vi "TCS_CFN_VS50BR_v1.vi"() -> ()   [LabVIEW 2017]
uses:
  <vilib>/Instr/_visa.llb/VISA Configure Serial Port (Instr).vi
panel:
  in  "Tab Control 4":enum32{"TCS_Utility", "TCS_Utility 2"}(tab)
  in  "Fact Reserved":bool
  in  "Download":bool
  in  "Fact Config":bool
  in  "NavOn":bool
  in  "Init":bool
  out "Half Second":bool[][](array[boolean])=[[FALSE, FALSE, FALSE, FALSE, FALSE, FALSE, FALSE, FALSE, FALSE, FALSE], [FALSE, FALSE, TRUE, TRUE, TRUE, TRUE, TRUE, FALSE, FALSE, FALSE], [FALSE, TRUE, FALSE, FALSE, FALSE, FALSE, FALSE, TRUE, FALSE, FALSE], [FALSE, TRUE, FALSE, FALSE, FALSE, FALSE, FALSE, TRUE, FALSE, FALSE], [FALSE, TRUE, FALSE, FALSE, FALSE, FALSE, FALSE, TRUE, FALSE, FALSE], [FALSE, TRUE, FALSE, FALSE, FALSE, FALSE, FALSE, TRUE, FALSE, FALSE], [FALSE, TRUE, FALSE, FALSE, FALSE, FALSE, FALSE, TRUE, FALSE, FALSE], [FALSE, TRUE, FALSE, FALSE, FALSE, FALSE, FALSE, TRUE, FALSE, FALSE], [FALSE, FALSE, TRUE, TRUE, TRUE, TRUE, TRUE, FALSE, FALSE, FALSE], [FALSE, FALSE, FALSE, FALSE, FALSE, FALSE, FALSE, FALSE, FALSE, FALSE]]
  out "Min 1":bool[][](array[boolean])=[[FALSE, FALSE, FALSE, FALSE, FALSE, FALSE, FALSE, FALSE, FALSE, FALSE], [FALSE, FALSE, TRUE, TRUE, TRUE, TRUE, TRUE, FALSE, FALSE, FALSE], [FALSE, TRUE, FALSE, FALSE, FALSE, FALSE, FALSE, TRUE, FALSE, FALSE], [FALSE, TRUE, FALSE, FALSE, FALSE, FALSE, FALSE, TRUE, FALSE, FALSE], [FALSE, TRUE, FALSE, FALSE, FALSE, FALSE, FALSE, TRUE, FALSE, FALSE], [FALSE, TRUE, FALSE, FALSE, FALSE, FALSE, FALSE, TRUE, FALSE, FALSE], [FALSE, TRUE, FALSE, FALSE, FALSE, FALSE, FALSE, TRUE, FALSE, FALSE], [FALSE, TRUE, FALSE, FALSE, FALSE, FALSE, FALSE, TRUE, FALSE, FALSE], [FALSE, FALSE, TRUE, TRUE, TRUE, TRUE, TRUE, FALSE, FALSE, FALSE], [FALSE, FALSE, FALSE, FALSE, FALSE, FALSE, FALSE, FALSE, FALSE, FALSE]]
  out "Min 0":bool[][](array[boolean])=[[FALSE, FALSE, FALSE, FALSE, FALSE, FALSE, FALSE, FALSE, FALSE, FALSE], [FALSE, FALSE, TRUE, TRUE, TRUE, TRUE, TRUE, FALSE, FALSE, FALSE], [FALSE, TRUE, FALSE, FALSE, FALSE, FALSE, FALSE, TRUE, FALSE, FALSE], [FALSE, TRUE, FALSE, FALSE, FALSE, FALSE, FALSE, TRUE, FALSE, FALSE], [FALSE, TRUE, FALSE, FALSE, FALSE, FALSE, FALSE, TRUE, FALSE, FALSE], [FALSE, TRUE, FALSE, FALSE, FALSE, FALSE, FALSE, TRUE, FALSE, FALSE], [FALSE, TRUE, FALSE, FALSE, FALSE, FALSE, FALSE, TRUE, FALSE, FALSE], [FALSE, TRUE, FALSE, FALSE, FALSE, FALSE, FALSE, TRUE, FALSE, FALSE], [FALSE, FALSE, TRUE, TRUE, TRUE, TRUE, TRUE, FALSE, FALSE, FALSE], [FALSE, FALSE, FALSE, FALSE, FALSE, FALSE, FALSE, FALSE, FALSE, FALSE]]
  out "Hour 1":bool[][](array[boolean])=[[FALSE, FALSE, FALSE, FALSE, FALSE, FALSE, FALSE, FALSE, FALSE, FALSE], [FALSE, FALSE, TRUE, TRUE, TRUE, TRUE, TRUE, FALSE, FALSE, FALSE], [FALSE, TRUE, FALSE, FALSE, FALSE, FALSE, FALSE, TRUE, FALSE, FALSE], [FALSE, TRUE, FALSE, FALSE, FALSE, FALSE, FALSE, TRUE, FALSE, FALSE], [FALSE, TRUE, FALSE, FALSE, FALSE, FALSE, FALSE, TRUE, FALSE, FALSE], [FALSE, TRUE, FALSE, FALSE, FALSE, FALSE, FALSE, TRUE, FALSE, FALSE], [FALSE, TRUE, FALSE, FALSE, FALSE, FALSE, FALSE, TRUE, FALSE, FALSE], [FALSE, TRUE, FALSE, FALSE, FALSE, FALSE, FALSE, TRUE, FALSE, FALSE], [FALSE, FALSE, TRUE, TRUE, TRUE, TRUE, TRUE, FALSE, FALSE, FALSE], [FALSE, FALSE, FALSE, FALSE, FALSE, FALSE, FALSE, FALSE, FALSE, FALSE]]
  out "Hour 0":bool[][](array[boolean])=[[FALSE, FALSE, FALSE, FALSE, FALSE, FALSE, FALSE, FALSE, FALSE, FALSE], [FALSE, FALSE, TRUE, TRUE, TRUE, TRUE, TRUE, FALSE, FALSE, FALSE], [FALSE, TRUE, FALSE, FALSE, FALSE, FALSE, FALSE, TRUE, FALSE, FALSE], [FALSE, TRUE, FALSE, FALSE, FALSE, FALSE, FALSE, TRUE, FALSE, FALSE], [FALSE, TRUE, FALSE, FALSE, FALSE, FALSE, FALSE, TRUE, FALSE, FALSE], [FALSE, TRUE, FALSE, FALSE, FALSE, FALSE, FALSE, TRUE, FALSE, FALSE], [FALSE, TRUE, FALSE, FALSE, FALSE, FALSE, FALSE, TRUE, FALSE, FALSE], [FALSE, TRUE, FALSE, FALSE, FALSE, FALSE, FALSE, TRUE, FALSE, FALSE], [FALSE, FALSE, TRUE, TRUE, TRUE, TRUE, TRUE, FALSE, FALSE, FALSE], [FALSE, FALSE, FALSE, FALSE, FALSE, FALSE, FALSE, FALSE, FALSE, FALSE]]
  in  "Stop":bool
  out "string in":string
  out "string out":string
  out "DV_Word":bool[](array[boolean])
  out "B_55":u8 format="%x"
  out "B_54":u8 format="%x"
  out "String":string
  in  "Send":bool
  in  "Tab Control":enum32{"Page 1", "Page 2", "Page 3"}(tab)
  in  "Offset Yaw":sgl(slide) scale=-180.0..180.0
  in  "Offset Roll":sgl(slide) scale=-180.0..180.0
  in  "Offset Pitch":sgl(slide) scale=-180.0..180.0
  in  "Longitude":sgl(slide)=-45.860622 scale=-180.0..180.0
  in  "Latitude":sgl(slide)=-23.213156 scale=-90.0..90.0
  in  "Azimuth":sgl(slide) scale=0.0..360.0
  in  "Height":sgl(slide)=622.367 scale=-2000.0..10000.0
  in  "LP_X-Up":sgl(slide) scale=-180.0..180.0
  in  "LP_Y-Easth":sgl(slide)=0.128098 scale=-180.0..180.0
  in  "LP_Z-North":sgl(slide)=0.467339 scale=-180.0..180.0
  # "B#55 (Configuration and Command Mode)"
  # "0x35"
  # "0xBD"
  # "0XFA"
  # "0XEE"
  # "0XAB"
  # "B#54 (Data Validity Word)"
  # "1= Installation Offset input valid data\n1= Launch Azimuth geodetic orientation, position, (lat, long, height) valid \n1= Velocity input valid data \nRFU\nRFU\nRFU\n 7,6     00= \"Init Cmd\" (Configuration parameters setting)\n           10= \"NAV_On\"\n           01= Reserved\n           11= Enter Configuration Mode"
  # "0\n1\n2\n3\n4\n5\n6\n7"
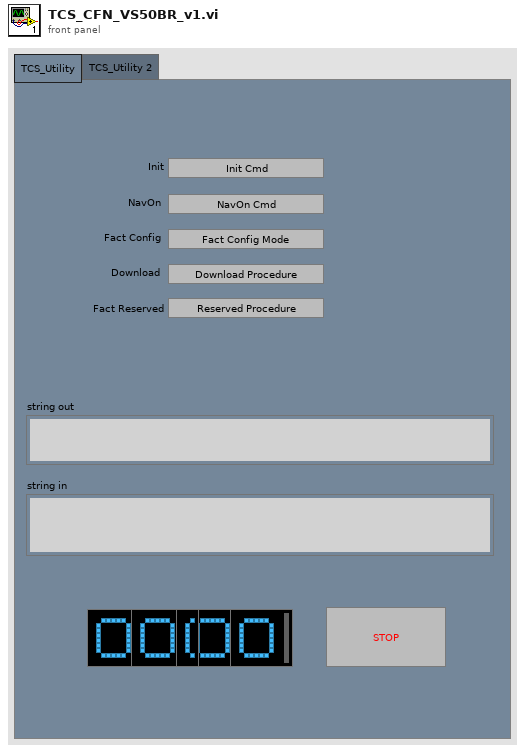
[diagram p1: front panel]
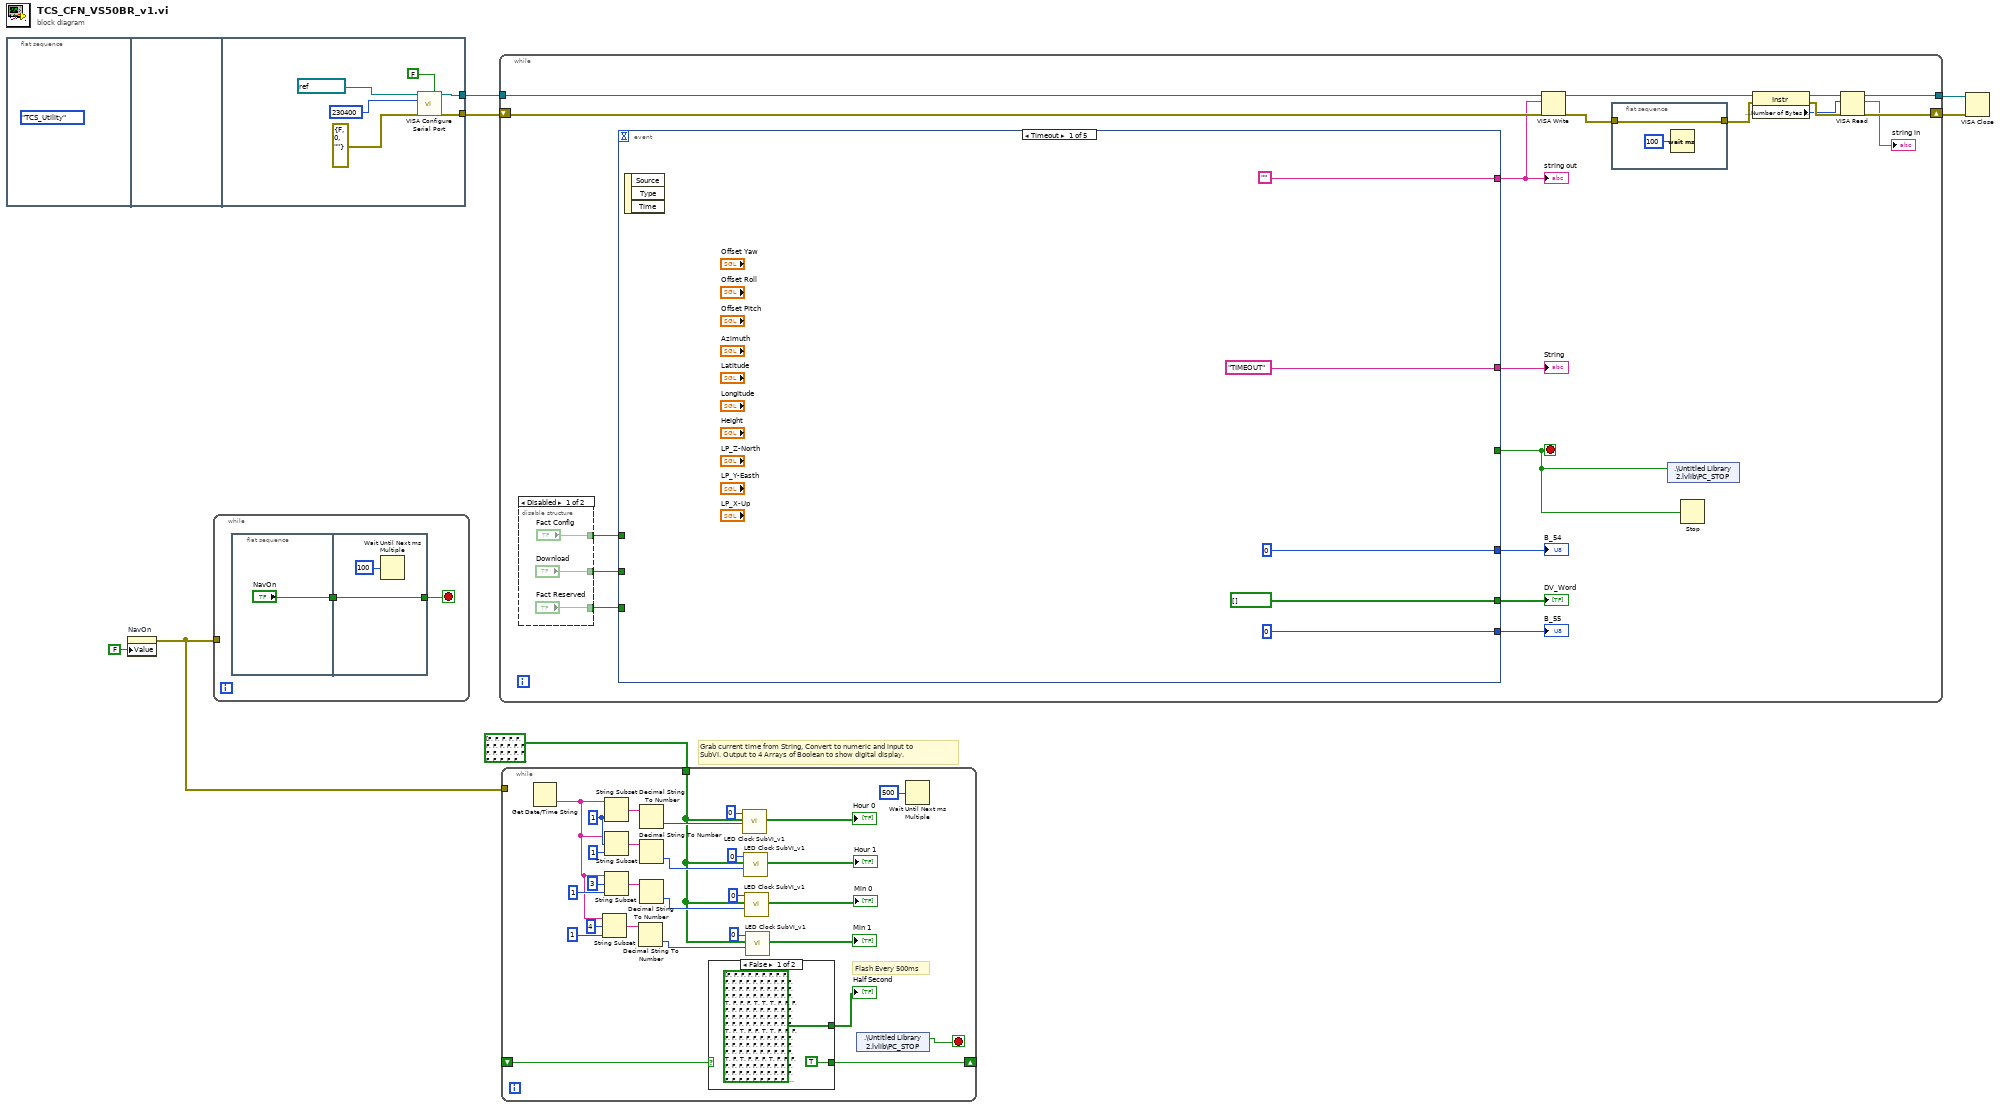
[diagram p0: block diagram]
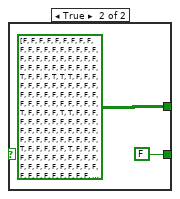
[diagram p2: hidden frame]
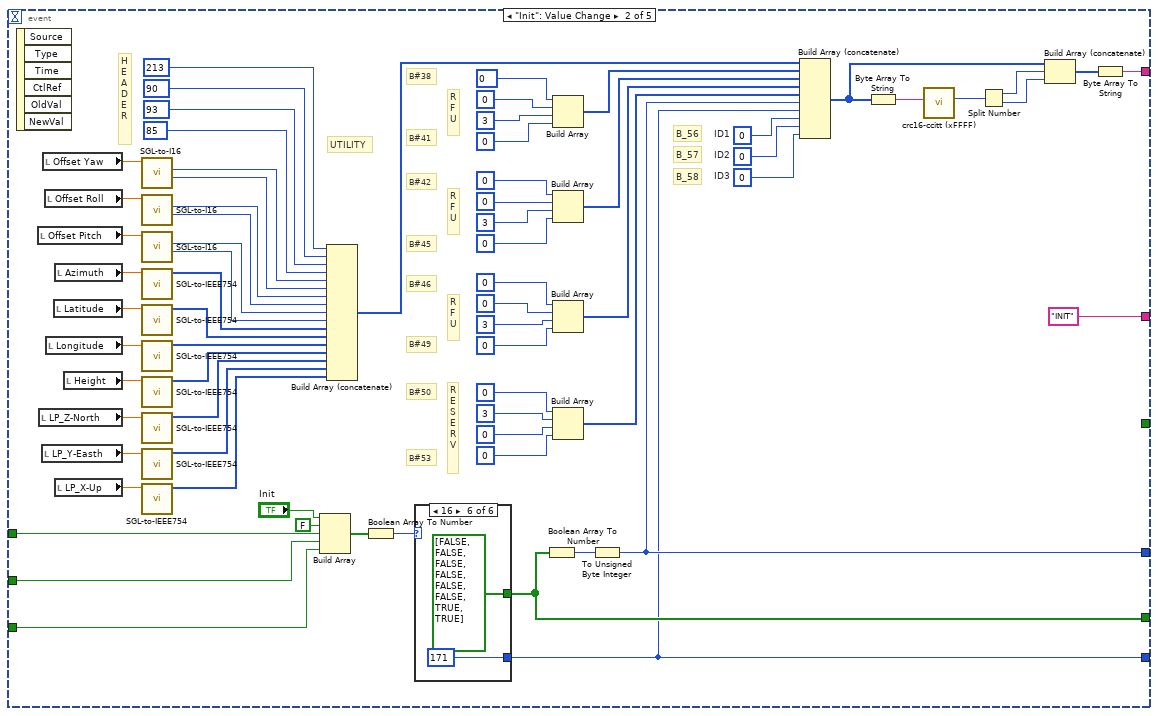
[diagram p3: hidden frame]
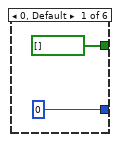
[diagram p4: hidden frame]
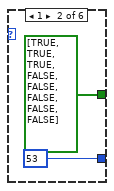
[diagram p5: hidden frame]
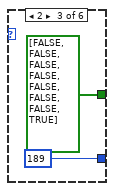
[diagram p6: hidden frame]
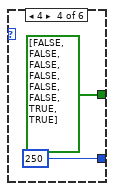
[diagram p7: hidden frame]
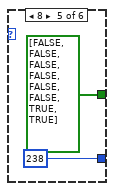
[diagram p8: hidden frame]
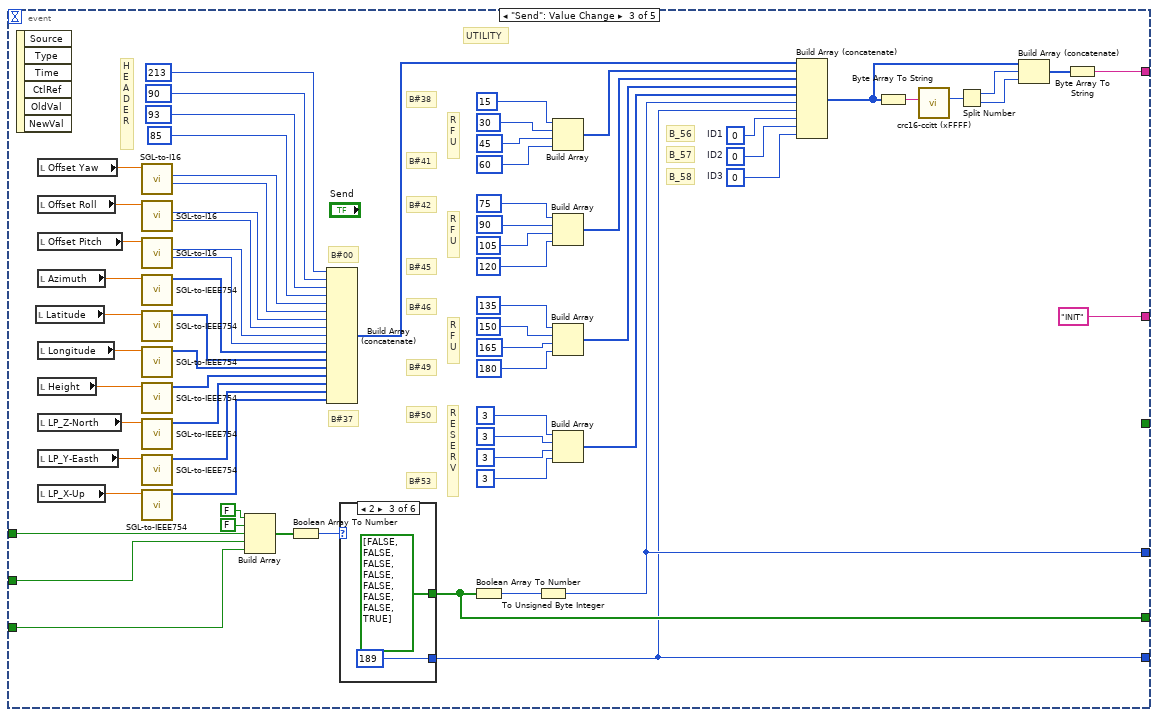
[diagram p9: hidden frame]
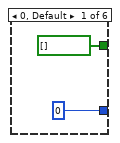
[diagram p10: hidden frame]
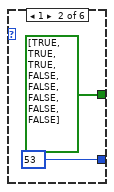
[diagram p11: hidden frame]
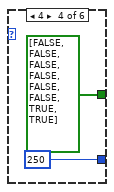
[diagram p12: hidden frame]
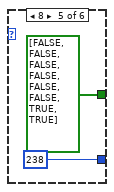
[diagram p13: hidden frame]
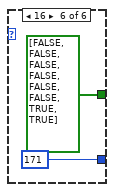
[diagram p14: hidden frame]
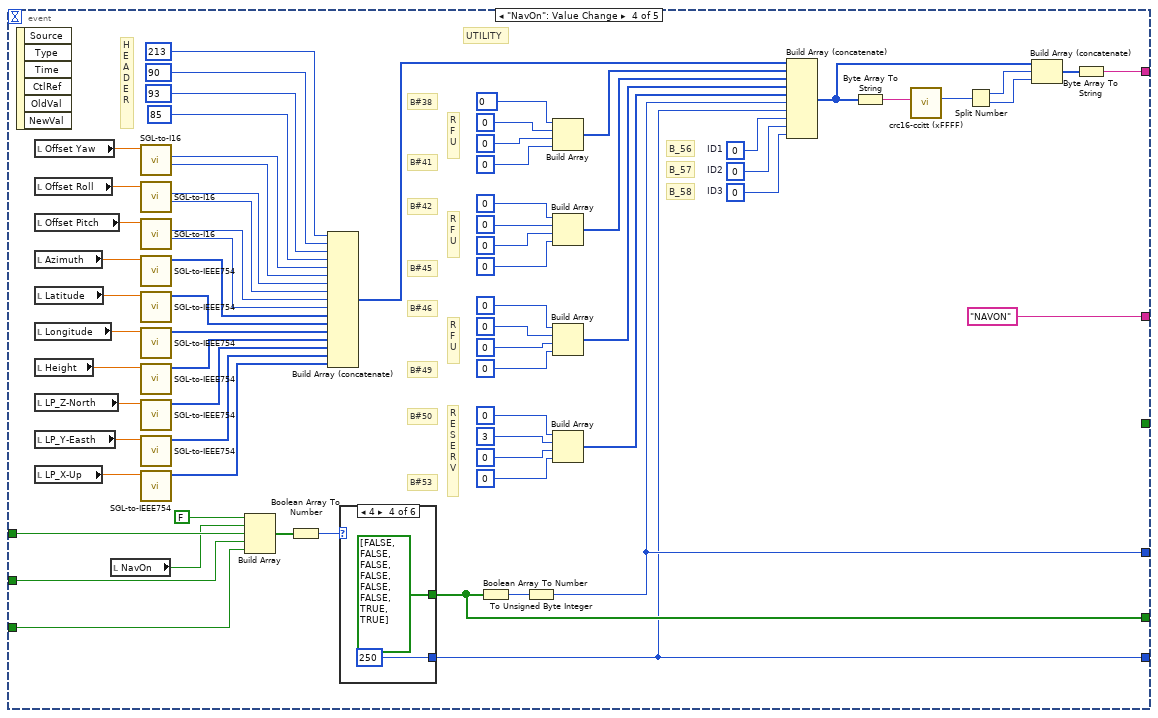
[diagram p15: hidden frame]
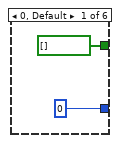
[diagram p16: hidden frame]
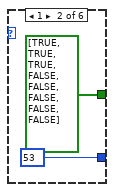
[diagram p17: hidden frame]
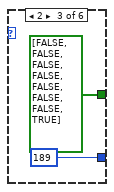
[diagram p18: hidden frame]
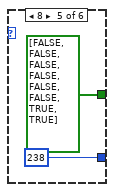
[diagram p19: hidden frame]
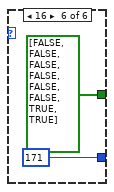
[diagram p20: hidden frame]
diagram:
  # "Grab current time from String, Convert to numeric and input to\nSubVI. Output to 4 Arrays of Boolean to show digital display."
  n1 = flat-sequence {
    tunnel: [w10] -> w7
    tunnel: [w9] -> w6
    frame #0 {
      (unwired) enum32{"TCS_Utility", "Parser"}."TCS_Utility" ("Tab Control 3")
    }
    frame #1 {
    }
    frame #2 {
      n2 = call-poly "VISA Configure Serial Port"("VISA resource name"=refnum<visa-resource-name> "COM4", "Enable Termination\nChar (T)"=FALSE ("Enable Termination\nChar (T)"), "baud rate (9600)"=u32 230400 ("Serial Settings:Baud Rate"), "error in (no error)"=errorcluster {"status"=FALSE, "code"=0, "source"=""}) -> ("VISA resource name out"=w10:refnum<visa-resource-name>, "error out"=w9:errorcluster)  [unwired: 10 in]
    }
  }
  n3 = property on="NavOn" class="Bool (strict)"("Value"=FALSE ("NavOn")) -> (error out=w1:errorcluster)  [unwired: 2 in, 1 out]
  n4 = while {
    tunnel: w1 -> [_]
    stop <- w15 stop-if-true
    n5 = flat-sequence {
      tunnel: ["NavOn"] -> w14
      tunnel: [w17] -> w15
      tunnel: w14 -> [w17]
      frame #0 {
      }
      frame #1 {
        n6 = Wait Until Next ms Multiple(millisecond multiple=u32 100) -> ()  [unwired: 1 out]
      }
    }
  }
  n7 = while {
    tunnel: w7 -> [w31]
    tunnel: [w21] -> w5
    shift-right: [w22] -> w4
    shift-left: w6 -> [w30]
    stop <- w19 stop-if-true
    n8 = disable-structure shown="Disabled" {
      disable-tunnel: ["Fact Config" _] -> w38
      disable-tunnel: ["Download" _] -> w37
      disable-tunnel: ["Fact Reserved" _] -> w36
      frame Disabled {
      }
      frame Enabled {
      }
    }
    n9 = event shown="[0] Timeout" {
      selector: _ -> [_ _ _ _ _]
      dyn-events: _ -> [_ _ _ _ _]
      timeout: _ -> [_ _ _ _ _]
      tunnel: ["" w66 w148 w230 ""] -> w29
      tunnel: w38 -> [_ w64 w146 w228 _]
      tunnel: w37 -> [_ w63 w145 w227 _]
      tunnel: w36 -> [_ w62 w144 w226 _]
      tunnel: [u8 0 w61 w143 w225 u8 0] -> w35
      tunnel: [bool[] [] ("DV_Word") w60 w142 w224 bool[] [] ("DV_Word")] -> w34
      tunnel: [u8 0 w56 w139 w223 u8 0] -> w33
      tunnel: [_ _ _ _ "Stop"] -> w19
      tunnel: ["TIMEOUT" "INIT" "INIT" "NAVON" "STOP"] -> w32
      event Timeout {
        n10 = event-data() -> ()  [unwired: 1 in, 3 out]
      }
      event "Init": Value Change {
        w72 = u8 0  # ID3
        w73 = u8 0  # ID2
        w74 = u8 0  # ID1
        # "B#53"
        # "B#50"
        # "B#49"
        # "B#46"
        # "B#45"
        # "B#42"
        # "B#41"
        # "B#38"
        # "B_58"
        # "B_57"
        # "B_56"
        # "R\nE\nS\nE\nR\nV"
        # "R\nF\nU"
        # "R\nF\nU"
        # "R\nF\nU"
        # "H\nE\nA\nD\nE\nR"
        # "UTILITY"
        n11 = event-data() -> ()  [unwired: 1 in, 6 out]
        n12 = local read "Offset Pitch"() -> (w53:sgl)
        n13 = local read "LP_Z-North"() -> (w48:sgl)
        n14 = local read "LP_Y-Easth"() -> (w47:sgl)
        n15 = local read "Offset Yaw"() -> (w55:sgl)
        n16 = local read "Offset Roll"() -> (w54:sgl)
        n17 = local read "Longitude"() -> (w50:sgl)
        n18 = local read "Latitude"() -> (w51:sgl)
        n19 = local read "Azimuth"() -> (w52:sgl)
        n20 = local read "LP_X-Up"() -> (w46:sgl)
        n21 = local read "Height"() -> (w49:sgl)
        n22 = call "SGL-to-I16.vi"("Range"=w55) -> ("lo(x)"=w107:u8, "hi(x)"=w108:u8)  [unwired: 8 in, 1 out]
        n23 = call "SGL-to-I16.vi"("Range"=w54) -> ("lo(x)"=w105:u8, "hi(x)"=w106:u8)  [unwired: 8 in, 1 out]
        n24 = call "SGL-to-I16.vi"("Range"=w53) -> ("lo(x)"=w103:u8, "hi(x)"=w104:u8)  [unwired: 8 in, 1 out]
        n25 = call "SGL-to-IEEE754.vi"("Input_DBL"=w52) -> ("Output_U8"=w102:u8[])  [unwired: 10 in]
        n26 = call "SGL-to-IEEE754.vi"("Input_DBL"=w51) -> ("Output_U8"=w101:u8[])  [unwired: 10 in]
        n27 = call "SGL-to-IEEE754.vi"("Input_DBL"=w50) -> ("Output_U8"=w100:u8[])  [unwired: 10 in]
        n28 = call "SGL-to-IEEE754.vi"("Input_DBL"=w49) -> ("Output_U8"=w99:u8[])  [unwired: 10 in]
        n29 = call "SGL-to-IEEE754.vi"("Input_DBL"=w48) -> ("Output_U8"=w98:u8[])  [unwired: 10 in]
        n30 = call "SGL-to-IEEE754.vi"("Input_DBL"=w47) -> ("Output_U8"=w97:u8[])  [unwired: 10 in]
        n31 = call "SGL-to-IEEE754.vi"("Input_DBL"=w46) -> ("Output_U8"=w96:u8[])  [unwired: 10 in]
        n32 = Build Array("Init", FALSE ("element"), w64, w63, w62) -> (w114:bool[])
        n33 = Build Array (concatenate)(u8 213, u8 90, u8 93, u8 85, w108, w107, w106, w105, w104, w103, w102, w101, w100, w99, w98, w97, w96) -> (w79:u8[])
        n34 = Boolean Array To Number(Boolean array=w114) -> (number=w113:u32)
        n35 = case shown="16" w113 {
          tunnel: [u8 0 u8 53 u8 189 u8 250 u8 238 u8 171] -> w56
          tunnel: [bool[] [] ("DV_Word") bool[] [TRUE, TRUE, TRUE, FALSE, FALSE, FALSE, FALSE, FALSE] ("DV_Word") bool[] [FALSE, FALSE, FALSE, FALSE, FALSE, FALSE, FALSE, TRUE] ("DV_Word") bool[] [FALSE, FALSE, FALSE, FALSE, FALSE, FALSE, TRUE, TRUE] ("DV_Word") bool[] [FALSE, FALSE, FALSE, FALSE, FALSE, FALSE, TRUE, TRUE] ("DV_Word") bool[] [FALSE, FALSE, FALSE, FALSE, FALSE, FALSE, TRUE, TRUE] ("DV_Word")] -> w60
          frame 0, Default {
          }
          frame 1 {
          }
          frame 2 {
          }
          frame 4 {
          }
          frame 8 {
          }
          frame 16 {
          }
        }
        n36 = Boolean Array To Number(Boolean array=w60) -> (number=w115:u32)
        n37 = Build Array(u8 0, u8 0, u8 3, u8 0) -> (w78:u8[])
        n38 = Build Array(u8 0, u8 0, u8 3, u8 0) -> (w77:u8[])
        n39 = Build Array(u8 0, u8 0, u8 3, u8 0) -> (w76:u8[])
        n40 = Build Array(u8 0, u8 3, u8 0, u8 0) -> (w75:u8[])
        n41 = To Unsigned Byte Integer(number=w115) -> (unsigned 8bit integer=w61:u8)
        n42 = Build Array (concatenate)(w79, w78, w77, w76, w75, w61, w56, w74, w73, w72) -> (w69:u8[])
        n43 = Byte Array To String(unsigned byte array=w69) -> (string=w71:string)
        n44 = call "crc16-ccitt (xFFFF).vi"("Message"=w71) -> ("CRC"=w70:u16)  [unwired: 9 in, 1 out]
        n45 = Split Number(x=w70) -> (hi(x)=w68:u8, lo(x)=w67:u8)
        n46 = Build Array (concatenate)(w69, w68, w67) -> (w65:u8[])
        n47 = Byte Array To String(unsigned byte array=w65) -> (string=w66:string)
      }
      event "Send": Value Change {
        w154 = u8 0  # ID3
        w155 = u8 0  # ID2
        w156 = u8 0  # ID1
        # "B#53"
        # "B#50"
        # "B#49"
        # "B#46"
        # "B#45"
        # "B#42"
        # "B#41"
        # "B#38"
        # "B#37"
        # "B#00"
        # "B_58"
        # "B_57"
        # "B_56"
        # "R\nE\nS\nE\nR\nV"
        # "R\nF\nU"
        # "R\nF\nU"
        # "R\nF\nU"
        # "H\nE\nA\nD\nE\nR"
        # "UTILITY"
        n48 = event-data() -> ()  [unwired: 1 in, 6 out]
        n49 = local read "Latitude"() -> (w134:sgl)
        n50 = local read "Offset Yaw"() -> (w138:sgl)
        n51 = local read "Offset Roll"() -> (w137:sgl)
        n52 = local read "Offset Pitch"() -> (w136:sgl)
        n53 = local read "Azimuth"() -> (w135:sgl)
        n54 = local read "Longitude"() -> (w133:sgl)
        n55 = local read "Height"() -> (w132:sgl)
        n56 = local read "LP_Z-North"() -> (w131:sgl)
        n57 = local read "LP_Y-Easth"() -> (w130:sgl)
        n58 = local read "LP_X-Up"() -> (w129:sgl)
        n59 = call "SGL-to-I16.vi"("Range"=w138) -> ("lo(x)"=w189:u8, "hi(x)"=w190:u8)  [unwired: 8 in, 1 out]
        n60 = call "SGL-to-I16.vi"("Range"=w137) -> ("lo(x)"=w187:u8, "hi(x)"=w188:u8)  [unwired: 8 in, 1 out]
        n61 = call "SGL-to-I16.vi"("Range"=w136) -> ("lo(x)"=w185:u8, "hi(x)"=w186:u8)  [unwired: 8 in, 1 out]
        n62 = call "SGL-to-IEEE754.vi"("Input_DBL"=w135) -> ("Output_U8"=w184:u8[])  [unwired: 10 in]
        n63 = call "SGL-to-IEEE754.vi"("Input_DBL"=w134) -> ("Output_U8"=w183:u8[])  [unwired: 10 in]
        n64 = call "SGL-to-IEEE754.vi"("Input_DBL"=w133) -> ("Output_U8"=w182:u8[])  [unwired: 10 in]
        n65 = call "SGL-to-IEEE754.vi"("Input_DBL"=w132) -> ("Output_U8"=w181:u8[])  [unwired: 10 in]
        n66 = call "SGL-to-IEEE754.vi"("Input_DBL"=w131) -> ("Output_U8"=w180:u8[])  [unwired: 10 in]
        n67 = call "SGL-to-IEEE754.vi"("Input_DBL"=w130) -> ("Output_U8"=w179:u8[])  [unwired: 10 in]
        n68 = call "SGL-to-IEEE754.vi"("Input_DBL"=w129) -> ("Output_U8"=w178:u8[])  [unwired: 10 in]
        n69 = Build Array(FALSE ("element"), FALSE ("element"), w146, w145, w144) -> (w196:bool[])
        n70 = Boolean Array To Number(Boolean array=w196) -> (number=w195:u32)
        n71 = Build Array (concatenate)(u8 213, u8 90, u8 93, u8 85, w190, w189, w188, w187, w186, w185, w184, w183, w182, w181, w180, w179, w178) -> (w161:u8[])
        n72 = case shown="2" w195 {
          tunnel: [u8 0 u8 53 u8 189 u8 250 u8 238 u8 171] -> w139
          tunnel: [bool[] [] ("DV_Word") bool[] [TRUE, TRUE, TRUE, FALSE, FALSE, FALSE, FALSE, FALSE] ("DV_Word") bool[] [FALSE, FALSE, FALSE, FALSE, FALSE, FALSE, FALSE, TRUE] ("DV_Word") bool[] [FALSE, FALSE, FALSE, FALSE, FALSE, FALSE, TRUE, TRUE] ("DV_Word") bool[] [FALSE, FALSE, FALSE, FALSE, FALSE, FALSE, TRUE, TRUE] ("DV_Word") bool[] [FALSE, FALSE, FALSE, FALSE, FALSE, FALSE, TRUE, TRUE] ("DV_Word")] -> w142
          frame 0, Default {
          }
          frame 1 {
          }
          frame 2 {
          }
          frame 4 {
          }
          frame 8 {
          }
          frame 16 {
          }
        }
        n73 = Boolean Array To Number(Boolean array=w142) -> (number=w197:u32)
        n74 = To Unsigned Byte Integer(number=w197) -> (unsigned 8bit integer=w143:u8)
        n75 = Build Array(u8 15, u8 30, u8 45, u8 60) -> (w160:u8[])
        n76 = Build Array(u8 75, u8 90, u8 105, u8 120) -> (w159:u8[])
        n77 = Build Array(u8 135, u8 150, u8 165, u8 180) -> (w158:u8[])
        n78 = Build Array(u8 3, u8 3, u8 3, u8 3) -> (w157:u8[])
        n79 = Build Array (concatenate)(w161, w160, w159, w158, w157, w143, w139, w156, w155, w154) -> (w151:u8[])
        n80 = Byte Array To String(unsigned byte array=w151) -> (string=w153:string)
        n81 = call "crc16-ccitt (xFFFF).vi"("Message"=w153) -> ("CRC"=w152:u16)  [unwired: 9 in, 1 out]
        n82 = Split Number(x=w152) -> (hi(x)=w150:u8, lo(x)=w149:u8)
        n83 = Build Array (concatenate)(w151, w150, w149) -> (w147:u8[])
        n84 = Byte Array To String(unsigned byte array=w147) -> (string=w148:string)
      }
      event "NavOn": Value Change {
        w236 = u8 0  # ID3
        w237 = u8 0  # ID2
        w238 = u8 0  # ID1
        # "B#53"
        # "B#50"
        # "B#49"
        # "B#46"
        # "B#45"
        # "B#42"
        # "B#41"
        # "B#38"
        # "B_58"
        # "B_57"
        # "B_56"
        # "R\nE\nS\nE\nR\nV"
        # "R\nF\nU"
        # "R\nF\nU"
        # "R\nF\nU"
        # "H\nE\nA\nD\nE\nR"
        # "UTILITY"
        n85 = event-data() -> ()  [unwired: 1 in, 6 out]
        n86 = local read "Offset Yaw"() -> (w220:sgl)
        n87 = local read "Offset Roll"() -> (w219:sgl)
        n88 = local read "Offset Pitch"() -> (w218:sgl)
        n89 = local read "Azimuth"() -> (w217:sgl)
        n90 = local read "Latitude"() -> (w216:sgl)
        n91 = local read "Longitude"() -> (w215:sgl)
        n92 = local read "Height"() -> (w214:sgl)
        n93 = local read "LP_Z-North"() -> (w213:sgl)
        n94 = local read "LP_Y-Easth"() -> (w212:sgl)
        n95 = local read "LP_X-Up"() -> (w211:sgl)
        n96 = local read "NavOn"() -> (w210:bool)
        n97 = call "SGL-to-I16.vi"("Range"=w220) -> ("lo(x)"=w271:u8, "hi(x)"=w272:u8)  [unwired: 8 in, 1 out]
        n98 = call "SGL-to-I16.vi"("Range"=w219) -> ("lo(x)"=w269:u8, "hi(x)"=w270:u8)  [unwired: 8 in, 1 out]
        n99 = call "SGL-to-I16.vi"("Range"=w218) -> ("lo(x)"=w267:u8, "hi(x)"=w268:u8)  [unwired: 8 in, 1 out]
        n100 = call "SGL-to-IEEE754.vi"("Input_DBL"=w217) -> ("Output_U8"=w266:u8[])  [unwired: 10 in]
        n101 = call "SGL-to-IEEE754.vi"("Input_DBL"=w216) -> ("Output_U8"=w265:u8[])  [unwired: 10 in]
        n102 = call "SGL-to-IEEE754.vi"("Input_DBL"=w215) -> ("Output_U8"=w264:u8[])  [unwired: 10 in]
        n103 = call "SGL-to-IEEE754.vi"("Input_DBL"=w214) -> ("Output_U8"=w263:u8[])  [unwired: 10 in]
        n104 = call "SGL-to-IEEE754.vi"("Input_DBL"=w213) -> ("Output_U8"=w262:u8[])  [unwired: 10 in]
        n105 = call "SGL-to-IEEE754.vi"("Input_DBL"=w212) -> ("Output_U8"=w261:u8[])  [unwired: 10 in]
        n106 = call "SGL-to-IEEE754.vi"("Input_DBL"=w211) -> ("Output_U8"=w260:u8[])  [unwired: 10 in]
        n107 = Build Array(FALSE ("element"), w210, w228, w227, w226) -> (w278:bool[])
        n108 = Boolean Array To Number(Boolean array=w278) -> (number=w277:u32)
        n109 = Build Array (concatenate)(u8 213, u8 90, u8 93, u8 85, w272, w271, w270, w269, w268, w267, w266, w265, w264, w263, w262, w261, w260) -> (w243:u8[])
        n110 = case shown="4" w277 {
          tunnel: [u8 0 u8 53 u8 189 u8 250 u8 238 u8 171] -> w223
          tunnel: [bool[] [] ("DV_Word") bool[] [TRUE, TRUE, TRUE, FALSE, FALSE, FALSE, FALSE, FALSE] ("DV_Word") bool[] [FALSE, FALSE, FALSE, FALSE, FALSE, FALSE, FALSE, TRUE] ("DV_Word") bool[] [FALSE, FALSE, FALSE, FALSE, FALSE, FALSE, TRUE, TRUE] ("DV_Word") bool[] [FALSE, FALSE, FALSE, FALSE, FALSE, FALSE, TRUE, TRUE] ("DV_Word") bool[] [FALSE, FALSE, FALSE, FALSE, FALSE, FALSE, TRUE, TRUE] ("DV_Word")] -> w224
          frame 0, Default {
          }
          frame 1 {
          }
          frame 2 {
          }
          frame 4 {
          }
          frame 8 {
          }
          frame 16 {
          }
        }
        n111 = Boolean Array To Number(Boolean array=w224) -> (number=w279:u32)
        n112 = To Unsigned Byte Integer(number=w279) -> (unsigned 8bit integer=w225:u8)
        n113 = Build Array(u8 0, u8 0, u8 0, u8 0) -> (w242:u8[])
        n114 = Build Array(u8 0, u8 0, u8 0, u8 0) -> (w241:u8[])
        n115 = Build Array(u8 0, u8 0, u8 0, u8 0) -> (w240:u8[])
        n116 = Build Array(u8 0, u8 3, u8 0, u8 0) -> (w239:u8[])
        n117 = Build Array (concatenate)(w243, w242, w241, w240, w239, w225, w223, w238, w237, w236) -> (w233:u8[])
        n118 = Byte Array To String(unsigned byte array=w233) -> (string=w235:string)
        n119 = call "crc16-ccitt (xFFFF).vi"("Message"=w235) -> ("CRC"=w234:u16)  [unwired: 9 in, 1 out]
        n120 = Split Number(x=w234) -> (hi(x)=w232:u8, lo(x)=w231:u8)
        n121 = Build Array (concatenate)(w233, w232, w231) -> (w229:u8[])
        n122 = Byte Array To String(unsigned byte array=w229) -> (string=w230:string)
      }
      event "Stop": Value Change {
        n123 = event-data() -> ()  [unwired: 1 in, 6 out]
      }
    }
    "string out" <- w29
    "B_54" <- w35
    "DV_Word" <- w34
    "B_55" <- w33
    "String" <- w32
    n124 = VISA Write(VISA resource name=w31, write buffer=w29, error in (no error)=w30) -> (VISA resource name out=w28:refnum<visa-resource-name>, error out=w26:errorcluster)  [unwired: 1 out]
    n125 = flat-sequence {
      tunnel: [w39] -> w27
      tunnel: w26 -> [w39]
      frame #0 {
        n126 = Wait (ms)(milliseconds to wait=u32 100) -> ()  [unwired: 1 out]
      }
    }
    n127 = shared-variable ".\\Untitled Library 2.lvlib\\PC_STOP"(w19) -> ()  [unwired: 1 in, 1 out]
    n128 = Stop(stop? (T)=w19) -> ()
    n129 = property class="Instr"(reference=w28, error in=w27) -> (reference out=w25:refnum<visa-resource-name>, error out=w24:errorcluster, "Serial Settings:Number of Bytes at Serial Port"=w23:u32)
    n130 = VISA Read(VISA resource name=w25, byte count=w23, error in (no error)=w24) -> (VISA resource name out=w21:refnum<visa-resource-name>, read buffer=→"string in":string, error out=w22:errorcluster)  [unwired: 1 out]
  }
  n131 = while {
    tunnel: bool[][] [[FALSE, FALSE, FALSE, FALSE, FALSE, FALSE, FALSE, FALSE, FALSE, FALSE, FALSE, FALSE, FALSE, FALSE, FALSE, FALSE, FALSE, FALSE, FALSE, FALSE, FALSE, FALSE, FALSE, FALSE, FALSE, FALSE, FALSE, FALSE, FALSE, FALSE, FALSE, FALSE, FALSE, FALSE, FALSE, FALSE, FALSE, FALSE, FALSE, TRUE], [FALSE, FALSE, FALSE, TRUE, TRUE, TRUE, FALSE, FALSE, FALSE, FALSE, FALSE, FALSE, FALSE, FALSE, FALSE, FALSE, FALSE, FALSE, FALSE, FALSE, FALSE, FALSE, FALSE, FALSE, FALSE, FALSE, FALSE, FALSE, FALSE, FALSE, FALSE, FALSE, FALSE, FALSE, FALSE, FALSE, FALSE, FALSE, FALSE, TRUE], [FALSE, FALSE, FALSE, FALSE, TRUE, TRUE, FALSE, FALSE, FALSE, FALSE, FALSE, FALSE, FALSE, FALSE, FALSE, FALSE, FALSE, FALSE, FALSE, FALSE, FALSE, FALSE, FALSE, FALSE, FALSE, FALSE, FALSE, FALSE, FALSE, FALSE, FALSE, FALSE, FALSE, FALSE, FALSE, FALSE, FALSE, FALSE, FALSE, TRUE], [FALSE, FALSE, FALSE, FALSE, FALSE, TRUE, FALSE, FALSE, FALSE, FALSE, FALSE, FALSE, FALSE, FALSE, FALSE, FALSE, FALSE, FALSE, FALSE, FALSE, FALSE, FALSE, FALSE, FALSE, FALSE, FALSE, FALSE, FALSE, FALSE, FALSE, FALSE, FALSE, FALSE, FALSE, FALSE, FALSE, FALSE, FALSE, FALSE, TRUE], [FALSE, FALSE, FALSE, FALSE, FALSE, TRUE, FALSE, FALSE, FALSE, FALSE, FALSE, FALSE, FALSE, FALSE, FALSE, FALSE, FALSE, FALSE, FALSE, FALSE, FALSE, FALSE, FALSE, FALSE, FALSE, FALSE, FALSE, FALSE, FALSE, FALSE, FALSE, FALSE, FALSE, FALSE, FALSE, FALSE, FALSE, FALSE, FALSE, TRUE], [FALSE, FALSE, FALSE, FALSE, FALSE, TRUE, FALSE, FALSE, FALSE, FALSE, FALSE, FALSE, FALSE, FALSE, FALSE, FALSE, FALSE, FALSE, FALSE, FALSE, FALSE, FALSE, FALSE, FALSE, FALSE, FALSE, FALSE, FALSE, FALSE, FALSE, FALSE, FALSE, FALSE, FALSE, FALSE, FALSE, FALSE, FALSE, FALSE, TRUE], [FALSE, FALSE, FALSE, FALSE, FALSE, TRUE, FALSE, FALSE, FALSE, FALSE, FALSE, FALSE, FALSE, FALSE, FALSE, FALSE, FALSE, FALSE, FALSE, FALSE, FALSE, FALSE, FALSE, FALSE, FALSE, FALSE, FALSE, FALSE, FALSE, FALSE, FALSE, FALSE, FALSE, FALSE, FALSE, FALSE, FALSE, FALSE, FALSE, TRUE], [FALSE, FALSE, FALSE, FALSE, FALSE, TRUE, FALSE, FALSE, FALSE, FALSE, FALSE, FALSE, FALSE, FALSE, FALSE, FALSE, FALSE, FALSE, FALSE, FALSE, FALSE, FALSE, FALSE, FALSE, FALSE, FALSE, FALSE, FALSE, FALSE, FALSE, FALSE, FALSE, FALSE, FALSE, FALSE, FALSE, FALSE, FALSE, FALSE, TRUE], [FALSE, FALSE, FALSE, TRUE, TRUE, TRUE, TRUE, TRUE, FALSE, FALSE, FALSE, FALSE, FALSE, FALSE, FALSE, FALSE, FALSE, FALSE, FALSE, FALSE, FALSE, FALSE, FALSE, FALSE, FALSE, FALSE, FALSE, FALSE, FALSE, FALSE, FALSE, FALSE, FALSE, FALSE, FALSE, FALSE, FALSE, FALSE, FALSE, TRUE], [FALSE, FALSE, FALSE, FALSE, FALSE, FALSE, FALSE, FALSE, FALSE, FALSE, FALSE, FALSE, FALSE, FALSE, FALSE, FALSE, FALSE, FALSE, FALSE, FALSE, FALSE, FALSE, FALSE, FALSE, FALSE, FALSE, FALSE, FALSE, FALSE, FALSE, FALSE, FALSE, FALSE, FALSE, FALSE, FALSE, FALSE, FALSE, FALSE, TRUE]] ("Base Array") -> [w306]
    shift-right: [w302] -> _
    shift-left: _ -> [w303]
    tunnel: w1 -> [_]
    stop <- w301 stop-if-true
    w319 = 1 ("length (rest)")
    # "Flash Every 500ms"
    n132 = Get Date/Time String() -> (time string=w311:string)  [unwired: 3 in, 1 out]
    n133 = String Subset(string=w311, offset (0)=4, length (rest)=1 ("length (rest)")) -> (substring=w308:string)
    n134 = String Subset(string=w311, offset (0)=3, length (rest)=1 ("length (rest)")) -> (substring=w314:string)
    n135 = String Subset(string=w311, length (rest)=w319) -> (substring=w321:string)  [unwired: 1 in]
    n136 = String Subset(string=w311, offset (0)=w319, length (rest)=1 ("length (rest)")) -> (substring=w316:string)
    n137 = Decimal String To Number(string=w308) -> (number=w307:i32)  [unwired: 2 in, 1 out]
    n138 = Decimal String To Number(string=w321) -> (number=w320:i32)  [unwired: 2 in, 1 out]
    n139 = Decimal String To Number(string=w316) -> (number=w315:i32)  [unwired: 2 in, 1 out]
    n140 = Decimal String To Number(string=w314) -> (number=w313:i32)  [unwired: 2 in, 1 out]
    n141 = case shown="False" w303 {
      tunnel: [bool[][] [[FALSE, FALSE, FALSE, FALSE, FALSE, FALSE, FALSE, FALSE, FALSE, FALSE, FALSE, FALSE, FALSE, FALSE, FALSE, FALSE, FALSE, FALSE, FALSE, FALSE, FALSE, FALSE, FALSE, FALSE, FALSE, FALSE, FALSE, FALSE, FALSE, FALSE, FALSE, FALSE, FALSE, FALSE, FALSE, FALSE, FALSE, FALSE, FALSE, TRUE], [FALSE, FALSE, FALSE, TRUE, TRUE, TRUE, FALSE, FALSE, FALSE, FALSE, FALSE, FALSE, FALSE, FALSE, FALSE, FALSE, FALSE, FALSE, FALSE, FALSE, FALSE, FALSE, FALSE, FALSE, FALSE, FALSE, FALSE, FALSE, FALSE, FALSE, FALSE, FALSE, FALSE, FALSE, FALSE, FALSE, FALSE, FALSE, FALSE, TRUE], [FALSE, TRUE, FALSE, FALSE, TRUE, TRUE, FALSE, FALSE, FALSE, FALSE, FALSE, FALSE, FALSE, FALSE, FALSE, FALSE, FALSE, FALSE, FALSE, FALSE, FALSE, FALSE, FALSE, FALSE, FALSE, FALSE, FALSE, FALSE, FALSE, FALSE, FALSE, FALSE, FALSE, FALSE, FALSE, FALSE, FALSE, FALSE, FALSE, TRUE], [FALSE, TRUE, FALSE, FALSE, FALSE, TRUE, FALSE, FALSE, FALSE, FALSE, FALSE, FALSE, FALSE, FALSE, FALSE, FALSE, FALSE, FALSE, FALSE, FALSE, FALSE, FALSE, FALSE, FALSE, FALSE, FALSE, FALSE, FALSE, FALSE, FALSE, FALSE, FALSE, FALSE, FALSE, FALSE, FALSE, FALSE, FALSE, FALSE, TRUE], [FALSE, FALSE, FALSE, FALSE, FALSE, TRUE, FALSE, FALSE, FALSE, FALSE, FALSE, FALSE, FALSE, FALSE, FALSE, FALSE, FALSE, FALSE, FALSE, FALSE, FALSE, FALSE, FALSE, FALSE, FALSE, FALSE, FALSE, FALSE, FALSE, FALSE, FALSE, FALSE, FALSE, FALSE, FALSE, FALSE, FALSE, FALSE, FALSE, TRUE], [FALSE, FALSE, FALSE, FALSE, FALSE, TRUE, FALSE, FALSE, FALSE, FALSE, FALSE, FALSE, FALSE, FALSE, FALSE, FALSE, FALSE, FALSE, FALSE, FALSE, FALSE, FALSE, FALSE, FALSE, FALSE, FALSE, FALSE, FALSE, FALSE, FALSE, FALSE, FALSE, FALSE, FALSE, FALSE, FALSE, FALSE, FALSE, FALSE, TRUE], [FALSE, TRUE, FALSE, FALSE, FALSE, TRUE, FALSE, FALSE, FALSE, FALSE, FALSE, FALSE, FALSE, FALSE, FALSE, FALSE, FALSE, FALSE, FALSE, FALSE, FALSE, FALSE, FALSE, FALSE, FALSE, FALSE, FALSE, FALSE, FALSE, FALSE, FALSE, FALSE, FALSE, FALSE, FALSE, FALSE, FALSE, FALSE, FALSE, TRUE], [FALSE, TRUE, FALSE, FALSE, FALSE, TRUE, FALSE, FALSE, FALSE, FALSE, FALSE, FALSE, FALSE, FALSE, FALSE, FALSE, FALSE, FALSE, FALSE, FALSE, FALSE, FALSE, FALSE, FALSE, FALSE, FALSE, FALSE, FALSE, FALSE, FALSE, FALSE, FALSE, FALSE, FALSE, FALSE, FALSE, FALSE, FALSE, FALSE, TRUE], [FALSE, FALSE, FALSE, TRUE, TRUE, TRUE, TRUE, TRUE, FALSE, FALSE, FALSE, FALSE, FALSE, FALSE, FALSE, FALSE, FALSE, FALSE, FALSE, FALSE, FALSE, FALSE, FALSE, FALSE, FALSE, FALSE, FALSE, FALSE, FALSE, FALSE, FALSE, FALSE, FALSE, FALSE, FALSE, FALSE, FALSE, FALSE, FALSE, TRUE], [FALSE, FALSE, FALSE, FALSE, FALSE, FALSE, FALSE, FALSE, FALSE, FALSE, FALSE, FALSE, FALSE, FALSE, FALSE, FALSE, FALSE, FALSE, FALSE, FALSE, FALSE, FALSE, FALSE, FALSE, FALSE, FALSE, FALSE, FALSE, FALSE, FALSE, FALSE, FALSE, FALSE, FALSE, FALSE, FALSE, FALSE, FALSE, FALSE, TRUE]] ("Base Array 2") bool[][] [[FALSE, FALSE, FALSE, FALSE, FALSE, FALSE, FALSE, FALSE, FALSE, FALSE, FALSE, FALSE, FALSE, FALSE, FALSE, FALSE, FALSE, FALSE, FALSE, FALSE, FALSE, FALSE, FALSE, FALSE, FALSE, FALSE, FALSE, FALSE, FALSE, FALSE, FALSE, FALSE, FALSE, FALSE, FALSE, FALSE, FALSE, FALSE, FALSE, TRUE], [FALSE, FALSE, FALSE, TRUE, TRUE, TRUE, FALSE, FALSE, FALSE, FALSE, FALSE, FALSE, FALSE, FALSE, FALSE, FALSE, FALSE, FALSE, FALSE, FALSE, FALSE, FALSE, FALSE, FALSE, FALSE, FALSE, FALSE, FALSE, FALSE, FALSE, FALSE, FALSE, FALSE, FALSE, FALSE, FALSE, FALSE, FALSE, FALSE, TRUE], [FALSE, FALSE, FALSE, FALSE, TRUE, TRUE, FALSE, FALSE, FALSE, FALSE, FALSE, FALSE, FALSE, FALSE, FALSE, FALSE, FALSE, FALSE, FALSE, FALSE, FALSE, FALSE, FALSE, FALSE, FALSE, FALSE, FALSE, FALSE, FALSE, FALSE, FALSE, FALSE, FALSE, FALSE, FALSE, FALSE, FALSE, FALSE, FALSE, TRUE], [FALSE, FALSE, FALSE, FALSE, FALSE, TRUE, FALSE, FALSE, FALSE, FALSE, FALSE, FALSE, FALSE, FALSE, FALSE, FALSE, FALSE, FALSE, FALSE, FALSE, FALSE, FALSE, FALSE, FALSE, FALSE, FALSE, FALSE, FALSE, FALSE, FALSE, FALSE, FALSE, FALSE, FALSE, FALSE, FALSE, FALSE, FALSE, FALSE, TRUE], [FALSE, FALSE, FALSE, FALSE, FALSE, TRUE, FALSE, FALSE, FALSE, FALSE, FALSE, FALSE, FALSE, FALSE, FALSE, FALSE, FALSE, FALSE, FALSE, FALSE, FALSE, FALSE, FALSE, FALSE, FALSE, FALSE, FALSE, FALSE, FALSE, FALSE, FALSE, FALSE, FALSE, FALSE, FALSE, FALSE, FALSE, FALSE, FALSE, TRUE], [FALSE, FALSE, FALSE, FALSE, FALSE, TRUE, FALSE, FALSE, FALSE, FALSE, FALSE, FALSE, FALSE, FALSE, FALSE, FALSE, FALSE, FALSE, FALSE, FALSE, FALSE, FALSE, FALSE, FALSE, FALSE, FALSE, FALSE, FALSE, FALSE, FALSE, FALSE, FALSE, FALSE, FALSE, FALSE, FALSE, FALSE, FALSE, FALSE, TRUE], [FALSE, FALSE, FALSE, FALSE, FALSE, TRUE, FALSE, FALSE, FALSE, FALSE, FALSE, FALSE, FALSE, FALSE, FALSE, FALSE, FALSE, FALSE, FALSE, FALSE, FALSE, FALSE, FALSE, FALSE, FALSE, FALSE, FALSE, FALSE, FALSE, FALSE, FALSE, FALSE, FALSE, FALSE, FALSE, FALSE, FALSE, FALSE, FALSE, TRUE], [FALSE, FALSE, FALSE, FALSE, FALSE, TRUE, FALSE, FALSE, FALSE, FALSE, FALSE, FALSE, FALSE, FALSE, FALSE, FALSE, FALSE, FALSE, FALSE, FALSE, FALSE, FALSE, FALSE, FALSE, FALSE, FALSE, FALSE, FALSE, FALSE, FALSE, FALSE, FALSE, FALSE, FALSE, FALSE, FALSE, FALSE, FALSE, FALSE, TRUE], [FALSE, FALSE, FALSE, TRUE, TRUE, TRUE, TRUE, TRUE, FALSE, FALSE, FALSE, FALSE, FALSE, FALSE, FALSE, FALSE, FALSE, FALSE, FALSE, FALSE, FALSE, FALSE, FALSE, FALSE, FALSE, FALSE, FALSE, FALSE, FALSE, FALSE, FALSE, FALSE, FALSE, FALSE, FALSE, FALSE, FALSE, FALSE, FALSE, TRUE], [FALSE, FALSE, FALSE, FALSE, FALSE, FALSE, FALSE, FALSE, FALSE, FALSE, FALSE, FALSE, FALSE, FALSE, FALSE, FALSE, FALSE, FALSE, FALSE, FALSE, FALSE, FALSE, FALSE, FALSE, FALSE, FALSE, FALSE, FALSE, FALSE, FALSE, FALSE, FALSE, FALSE, FALSE, FALSE, FALSE, FALSE, FALSE, FALSE, TRUE]] ("Base Array 2")] -> w304
      tunnel: [TRUE FALSE] -> w302
      frame False {
      }
      frame True {
      }
    }
    "Half Second" <- w304
    n142 = call "LED Clock SubVI_v1.vi"("Number"=w320, "Array"=w306, "Position"=0) -> ("Time Out"=→"Hour 0":bool[][])  [unwired: 8 in]
    n143 = call "LED Clock SubVI_v1.vi"("Number"=w315, "Array"=w306, "Position"=0) -> ("Time Out"=→"Hour 1":bool[][])  [unwired: 8 in]
    n144 = call "LED Clock SubVI_v1.vi"("Number"=w313, "Array"=w306, "Position"=0) -> ("Time Out"=→"Min 0":bool[][])  [unwired: 8 in]
    n145 = call "LED Clock SubVI_v1.vi"("Number"=w307, "Array"=w306, "Position"=0) -> ("Time Out"=→"Min 1":bool[][])  [unwired: 8 in]
    n146 = shared-variable ".\\Untitled Library 2.lvlib\\PC_STOP"() -> (w301:bool)  [unwired: 1 in, 1 out]
    n147 = Wait Until Next ms Multiple(millisecond multiple=u32 500) -> ()  [unwired: 1 out]
  }
  n148 = VISA Close(VISA resource name=w5, error in (no error)=w4) -> ()  [unwired: 1 out]
